vi "Convert_TrajectoryFile_To_PathWeaverJSON.vi"() -> ()   [LabVIEW 2019]
uses:
  <vilib>/Rock Robotics/WPI/ThirdParty/JAS_Junk/TrajLib/TypeDef/TRAJ_STATE.ctl
  <vilib>/Rock Robotics/WPI/ThirdParty/JAS_Junk/TrajLib/TypeDef/POSE2D.ctl
  <vilib>/Rock Robotics/WPI/ThirdParty/JAS_Junk/TrajLib/TypeDef/TRANSLATION2D.ctl
  <vilib>/Rock Robotics/WPI/ThirdParty/JAS_Junk/TrajLib/TypeDef/ROTATION2D.ctl
  <vilib>/Rock Robotics/WPI/ThirdParty/JAS_Junk/TrajLib/Trajectory_Library.lvlib
panel:
  in  "End Program":bool
  in  "Tab Control":T1(tab)
  in  "Trajectory CSV File":path
  in  "Read JSON Fiile":bool
  out "File Read Error":errorcluster
  in  "WheelBase":dbl=0.6
  out "Position":cluster{dbl[], dbl[]}[](graph)
  out "Trajectory Data":cluster{dbl[], dbl[]}[](graph)
  out "Traj States\nSize":i32
  out "Trajectory States":T2[](array[typedef]) {"POSE"."ROTATION"."SIN" format="%13.4f"; "POSE"."ROTATION"."COS" format="%13.4f"; "POSE"."ROTATION"."VALUE" format="%13.4f"; "POSE"."TRANSLATION"."Y" format="%14.3f"; "POSE"."TRANSLATION"."X" format="%14.3f"}
  in  "PathWeaver Length Units":T6(radio)
  out "File Saved\nWithout\nError":bool
  in  "Trajectory Type":enum32{"Radio Selection 1", "Radio Selection 2"}(radio)
  out "File Creation\nError":errorcluster
  in  "PathWeaver JSON File Name":path
  in  "CreateCmdList":bool
  out "Ready to\nWrite FIle":bool
  # "Convert trajectory CSV file to Pathweaver JSON file"
  # "Instructions: \n---------------- \nThis utility reads a trajectory CSV file,  The results are plotted for review.  \nThis file can then be written to a PathWeaver JSON file.\n\nNotes:\n---------\n - Pathweaver sets the Y orign at the top left.  This trajectory library utilties use the bottom right.  This utility converts the Y position value to be consistent. \n   There are no consequences when the trajectory is saved as a robot relative trajectory.  For absolute trajectories, the robot position needs to\n   condier this."
  # "Meters"
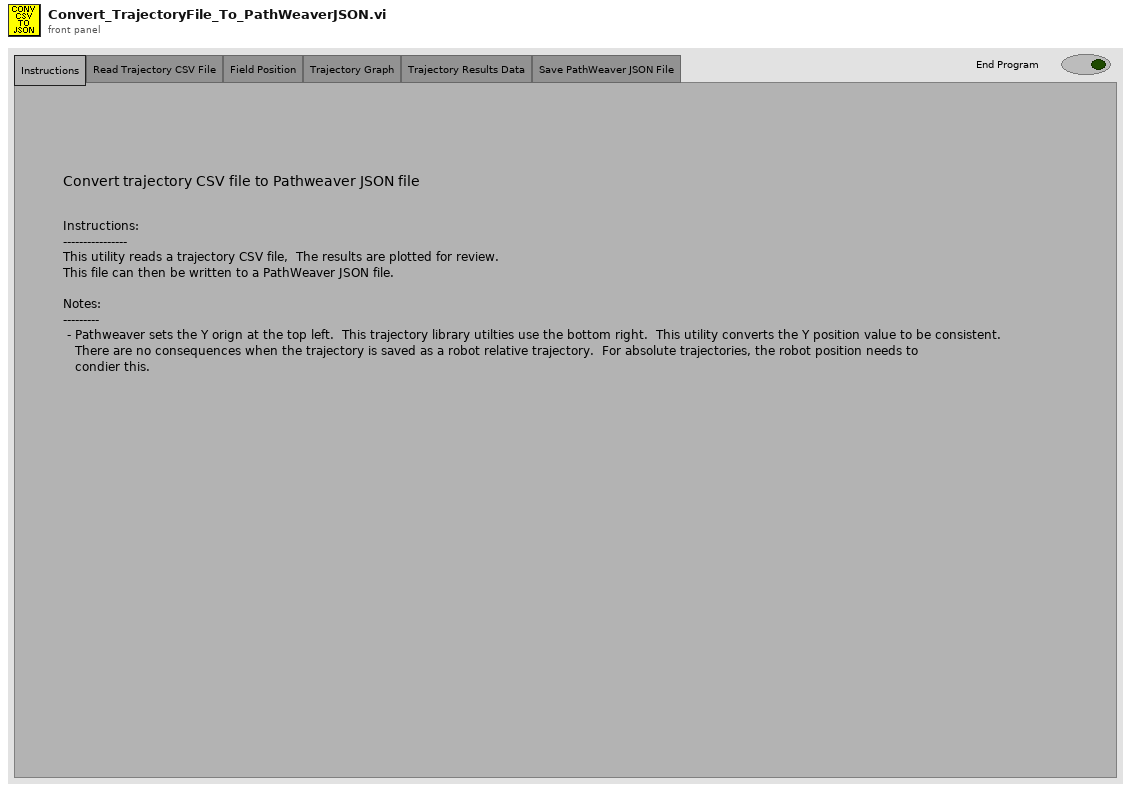
[diagram p1: front panel]
types:
  T1 = enum32{"Instructions", "Read Trajectory CSV File", "Field Position", "Trajectory Graph", "Trajectory Results Data", "Save PathWeaver JSON File"}
  T2 = typedef "Trajectory_Library.lvlib/TRAJ_STATE.ctl" = cluster{"TimeSeconds":dbl, "Velocity":dbl, "Acceleration":dbl, "POSE":T3, "Curvature":dbl}
  T3 = typedef "Trajectory_Library.lvlib/POSE2D.ctl" = cluster{"TRANSLATION":T4, "ROTATION":T5}
  T4 = typedef "Trajectory_Library.lvlib/TRANSLATION2D.ctl" = cluster{"X":dbl, "Y":dbl}
  T5 = typedef "Trajectory_Library.lvlib/ROTATION2D.ctl" = cluster{"VALUE":dbl, "COS":dbl, "SIN":dbl}
  T6 = enum32{"Radio Selection 1", "Radio Selection 2", "Radio Selection 3", "Radio Selection 4", "Radio Selection 5"}
  T7 = typedef "Trajectory_Library.lvlib/TRAJECTORY.ctl" = cluster{"TotalTImeSecs":dbl, "States":T2[]}
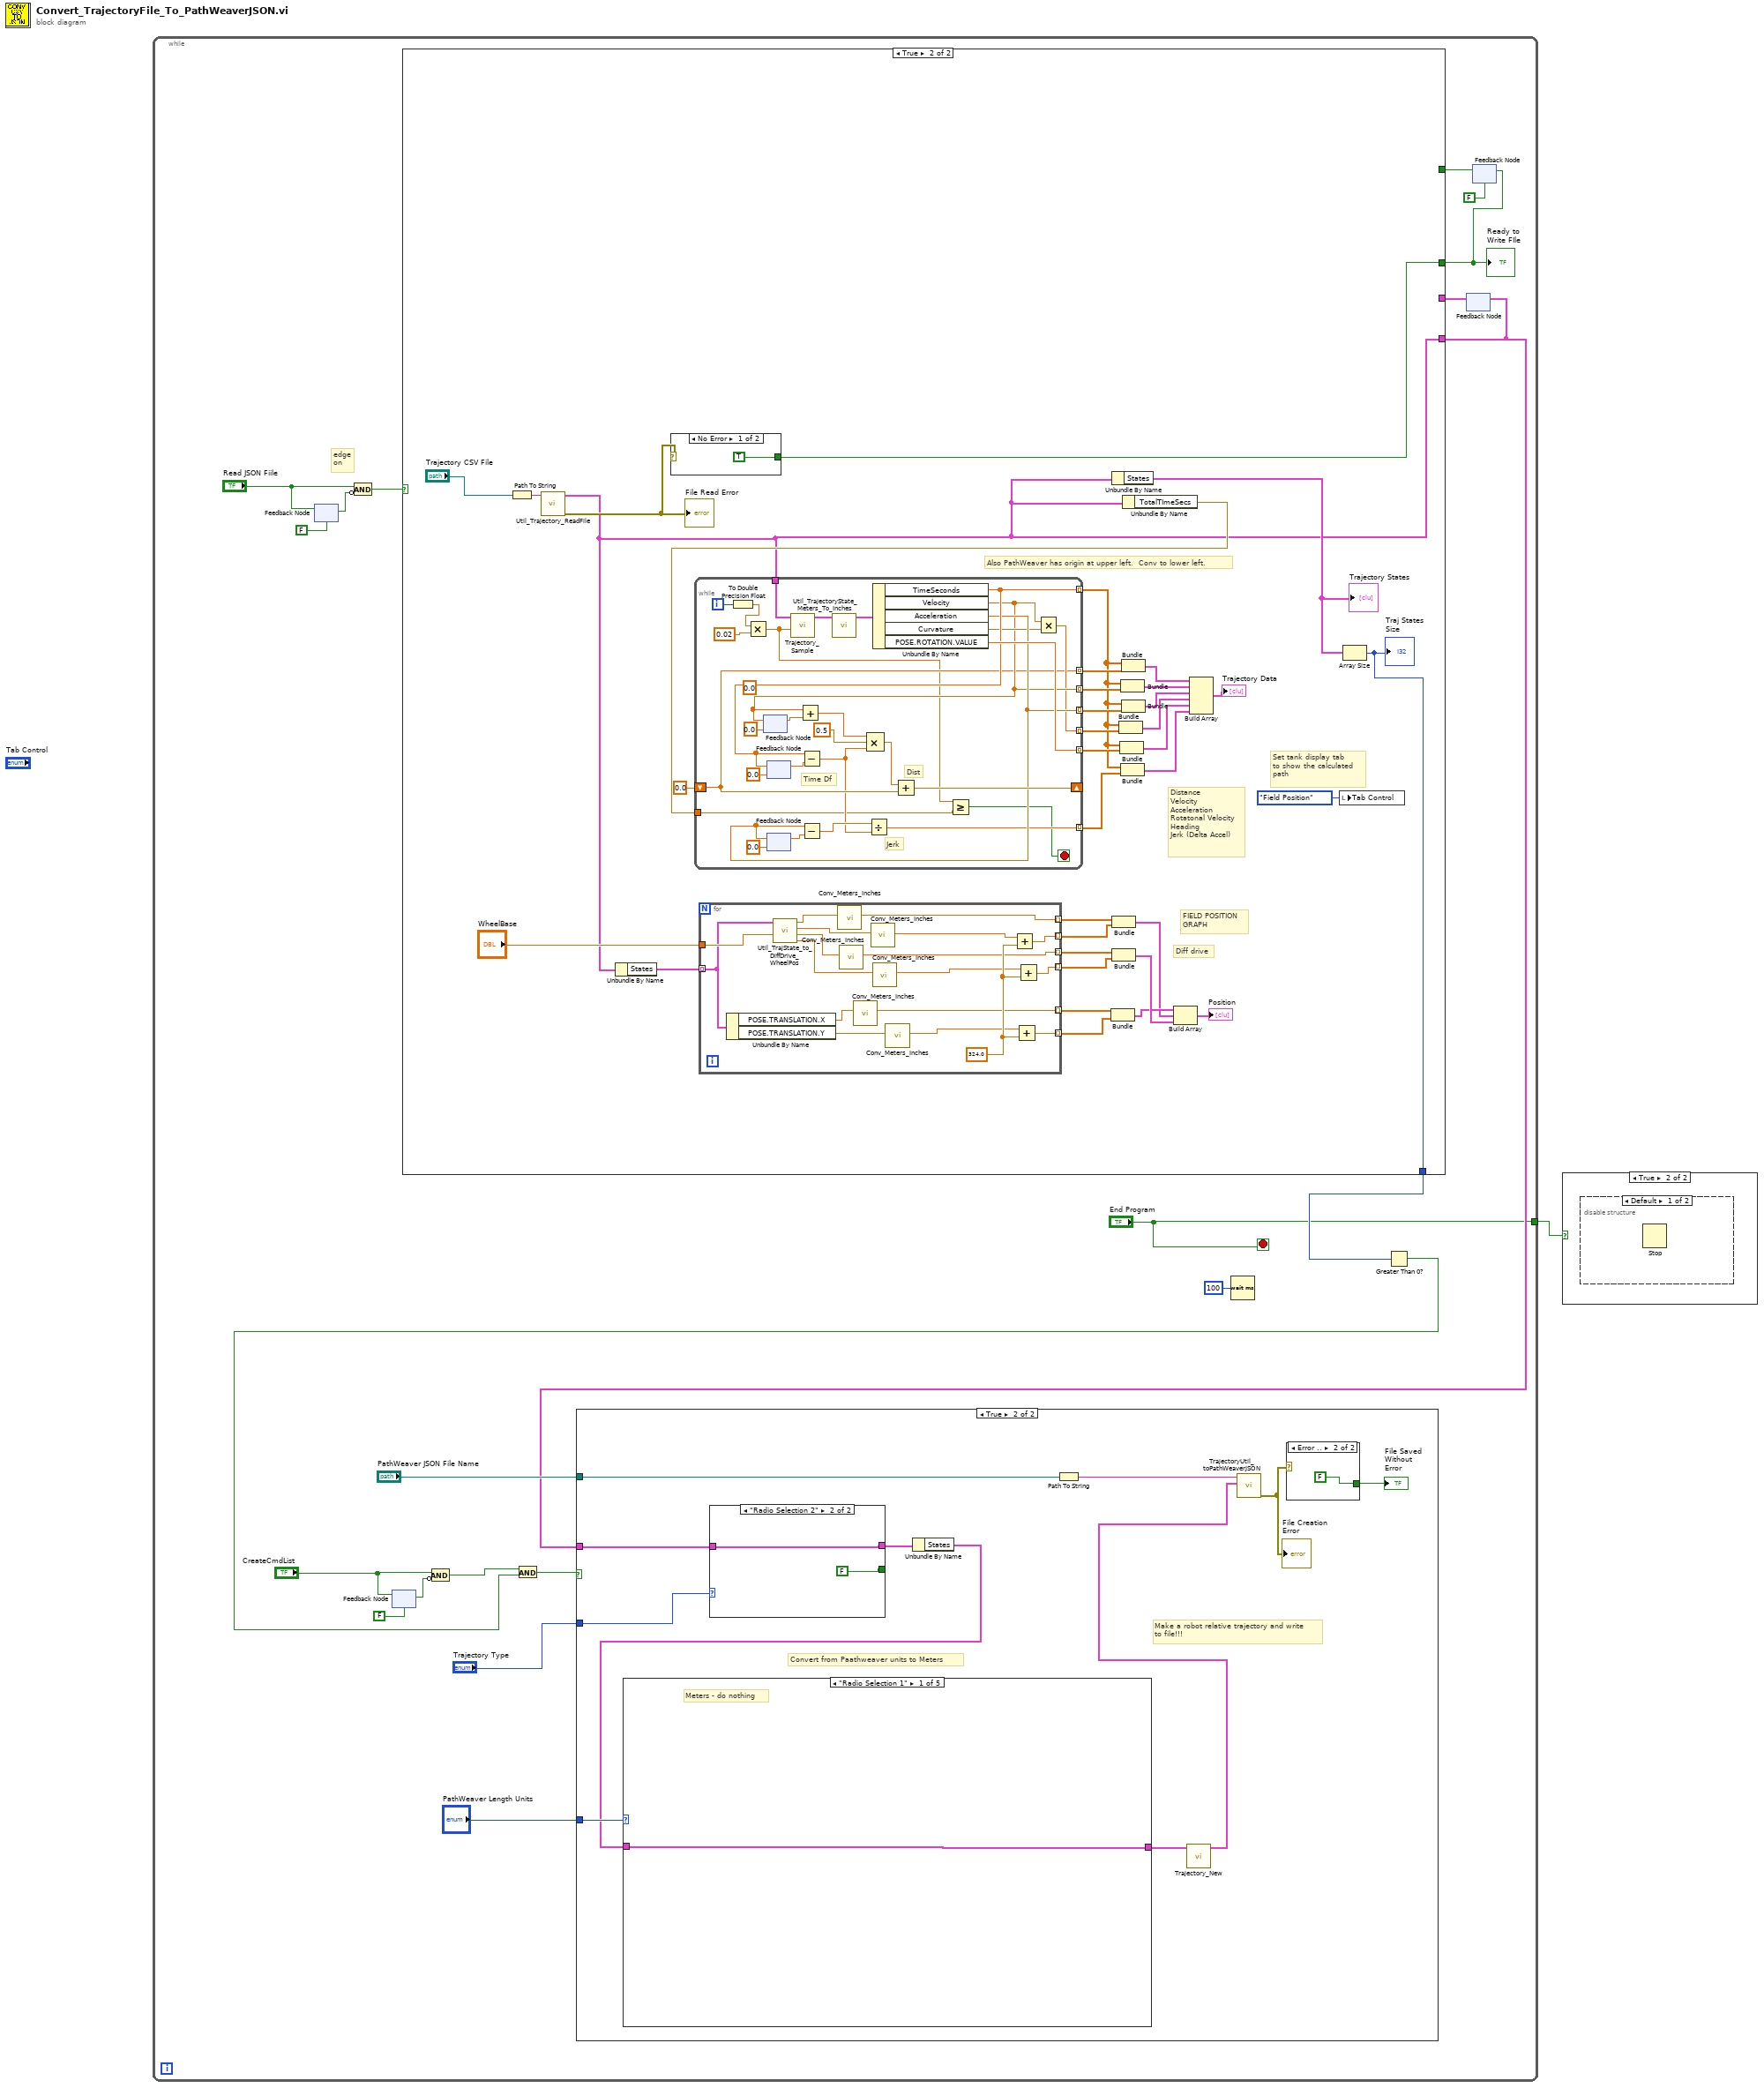
[diagram p0: block diagram]
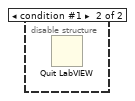
[diagram p3: hidden frame]
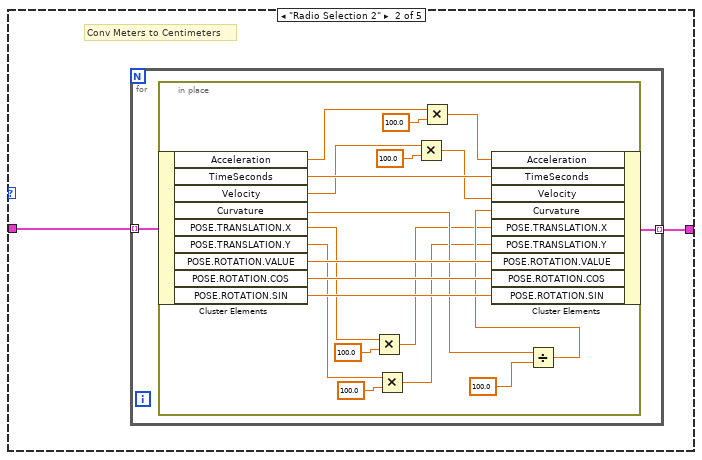
[diagram p5: hidden frame]
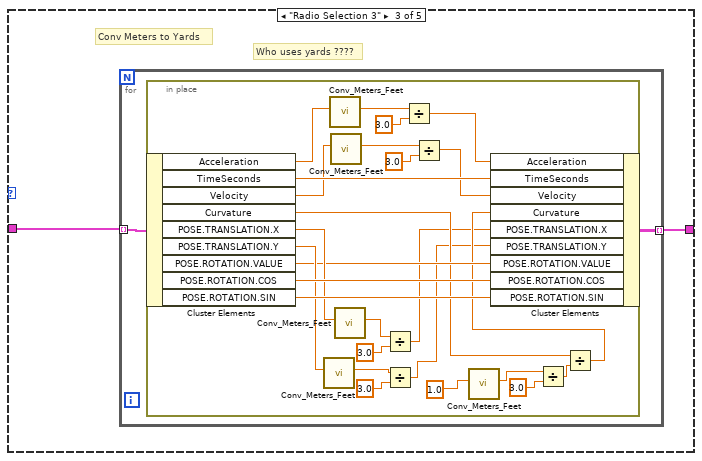
[diagram p6: hidden frame]
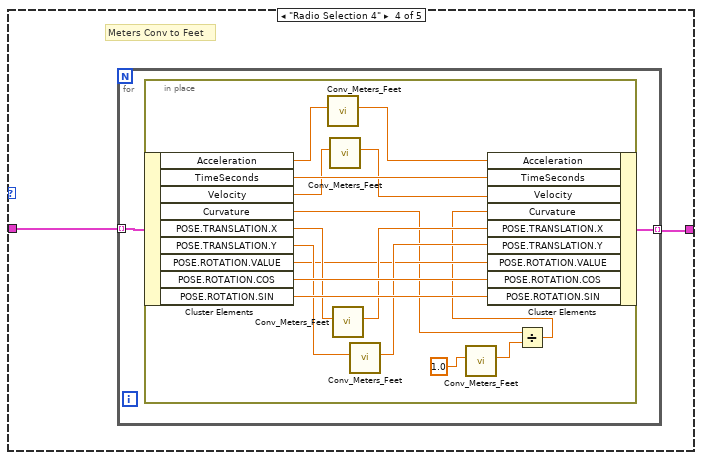
[diagram p7: hidden frame]
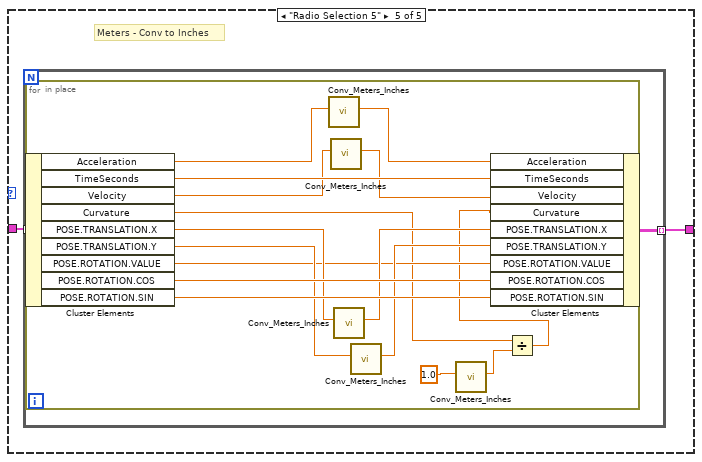
[diagram p8: hidden frame]
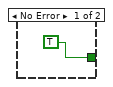
[diagram p9: hidden frame]
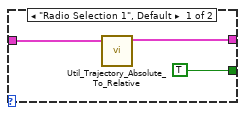
[diagram p10: hidden frame]
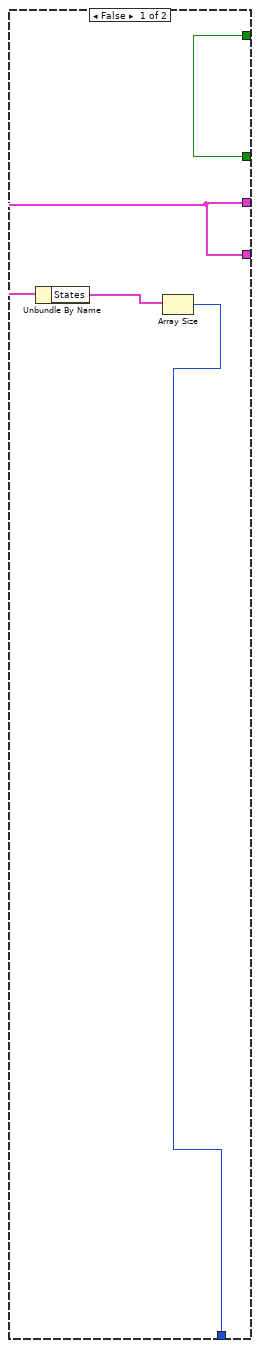
[diagram p11: hidden frame]
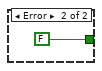
[diagram p12: hidden frame]
diagram:
  n1 = while {
    tunnel: ["End Program"] -> w1
    stop <- "End Program" stop-if-true
    # "edge\non"
    n2 = feedback #1(FALSE ("CreateCmdList")) -> (w12:bool)
    n3 = feedback-in #1("Read JSON Fiile") -> ()
    n4 = Compound Arithmetic op=AND("Read JSON Fiile", invert w12) -> (w10:bool)
    n5 = feedback-in #2("CreateCmdList") -> ()
    n6 = feedback #2(FALSE ("CreateCmdList")) -> (w15:bool)
    n7 = Compound Arithmetic op=AND("CreateCmdList", invert w15) -> (w14:bool)
    n8 = Wait (ms)(milliseconds to wait=u32 100) -> ()  [unwired: 1 out]
    n9 = feedback #3() -> (w21:T7)  [unwired: 1 in]
    n10 = feedback #4(FALSE) -> (w6:bool)
    n11 = case shown="True" w10 {
      tunnel: [w136 w139] -> w18
      tunnel: w21 -> [w136 _]
      tunnel: [w138 w174] -> w17
      tunnel: [w137 w172] -> w8
      tunnel: w6 -> [w137 _]
      frame False {
        n12 = Unbundle By Name(w136) -> ("States"=w135:T2[])
        n13 = Array Size(array=w135) -> (size(s)=w138:i32)
      }
      frame True {
        (unwired) 0.0
        # "Diff drive"
        # "FIELD POSITION\nGRAPH"
        # "Distance\nVelocity\nAcceleration\nRotatonal Velocity\nHeading\nJerk (Delta Accel)"
        # "Also PathWeaver has origin at upper left.  Conv to lower left."
        # "Set tank display tab\nto show the calculated\npath"
        n14 = Path To String(path="Trajectory CSV File") -> (string=w144:string)
        n15 = call <vilib>:"Util_Trajectory_ReadFile.vi"("FileName"=w144) -> ("error out"=w143:errorcluster, "outTRAJECTORY"=w139:T7)  [unwired: 8 in, 1 out]
        "File Read Error" <- w143
        n16 = Unbundle By Name(w139) -> ("States"=w145:T2[])
        n17 = case shown="No Error" w143 {
          tunnel: [TRUE FALSE] -> w172
          frame No Error {
          }
          frame Error {
          }
        }
        n18 = for {
          tunnel: w145 -> [w187] mode=indexing
          tunnel: "WheelBase" -> [w192]
          tunnel: [w181] -> w154 mode=indexing
          tunnel: [w183] -> w153 mode=indexing
          tunnel: [w179] -> w152 mode=indexing
          tunnel: [w182] -> w151 mode=indexing
          tunnel: [w176] -> w147 mode=indexing
          tunnel: [w177] -> w146 mode=indexing
          w184 = 324.0 ("y")
          n19 = Unbundle By Name(w187) -> ("POSE.TRANSLATION.X"=w186:dbl, "POSE.TRANSLATION.Y"=w185:dbl)
          n20 = call <vilib>:"Util_TrajState_to_DiffDrive_WheelPos.vi"("Wheelbase"=w192, "TRAJ_STATE"=w187) -> ("Right Y"=w188:dbl, "Right X"=w189:dbl, "Left Y"=w190:dbl, "Left X"=w191:dbl)  [unwired: 6 in]
          n21 = call <vilib>:"Conv_Meters_Inches.vi"("Meters"=w191) -> ("Inches"=w181:dbl)  [unwired: 10 in]
          n22 = call <vilib>:"Conv_Meters_Inches.vi"("Meters"=w189) -> ("Inches"=w179:dbl)  [unwired: 10 in]
          n23 = call <vilib>:"Conv_Meters_Inches.vi"("Meters"=w186) -> ("Inches"=w177:dbl)  [unwired: 10 in]
          n24 = call <vilib>:"Conv_Meters_Inches.vi"("Meters"=w190) -> ("Inches"=w180:dbl)  [unwired: 10 in]
          n25 = call <vilib>:"Conv_Meters_Inches.vi"("Meters"=w188) -> ("Inches"=w178:dbl)  [unwired: 10 in]
          n26 = call <vilib>:"Conv_Meters_Inches.vi"("Meters"=w185) -> ("Inches"=w175:dbl)  [unwired: 10 in]
          n27 = Add(x=w180, y=w184) -> (x+y=w183:dbl)
          n28 = Add(x=w175, y=w184) -> (x+y=w176:dbl)
          n29 = Add(x=w178, y=w184) -> (x+y=w182:dbl)
        }
        n30 = Bundle(w146, w147) -> (w149:cluster{dbl[], dbl[]})  [unwired: 1 in]
        n31 = Unbundle By Name(w139) -> ("States"=w140:T2[])
        "Trajectory States" <- w140
        n32 = Bundle(w154, w153) -> (w148:cluster{dbl[], dbl[]})  [unwired: 1 in]
        n33 = Bundle(w152, w151) -> (w150:cluster{dbl[], dbl[]})  [unwired: 1 in]
        n34 = Unbundle By Name(w139) -> ("TotalTImeSecs"=w156:dbl)
        n35 = while {
          tunnel: [w214] -> w158 mode=indexing
          tunnel: [w205] -> w168 mode=indexing
          tunnel: [w207] -> w167 mode=indexing
          tunnel: [w211] -> w166 mode=indexing
          tunnel: [w206] -> w165 mode=indexing
          tunnel: [w221] -> w164 mode=indexing
          shift-right: [w215] -> _
          shift-left: 0.0 -> [w205]
          tunnel: [w209] -> w157 mode=indexing
          tunnel: w156 -> [w201]
          tunnel: w139 -> [w199]
          i -> [w198]
          stop <- w200 stop-if-true
          # "Time Df"
          # "Jerk"
          # "Dist"
          n36 = To Double Precision Float(number=w198) -> (double precision float=w197:dbl)
          n37 = Multiply(x=w197, y=0.02) -> (x*y=w195:dbl)
          n38 = feedback #5(0.0 ("TimeSeconds")) -> (w217:dbl)
          n39 = feedback #6(0.0 ("TimeSeconds")) -> (w219:dbl)
          n40 = feedback #7(0.0 ("TimeSeconds")) -> (w212:dbl)
          n41 = call <vilib>:"Trajectory_Sample.vi"("Time"=w195, "InputTRAJECTORY"=w199) -> ("OutputTRAJ_STATE"=w193:T2)  [unwired: 9 in]
          n42 = call <vilib>:"Util_TrajectoryState_Meters_To_Inches.vi"("absTRAJECTORY"=w193) -> ("outputRelativeTRAJECTORY"=w194:T2)  [unwired: 10 in]
          n43 = Unbundle By Name(w194) -> ("TimeSeconds"=w214:dbl, "Velocity"=w207:dbl, "Acceleration"=w211:dbl, "Curvature"=w208:dbl, "POSE.ROTATION.VALUE"=w221:dbl)
          n44 = feedback-in #5(w207) -> ()
          n45 = feedback-in #6(w214) -> ()
          n46 = feedback-in #7(w211) -> ()
          n47 = Add(x=w207, y=w217) -> (x+y=w216:dbl)
          n48 = Subtract(x=w214, y=w219) -> (x-y=w202:dbl)
          n49 = Subtract(x=w211, y=w212) -> (x-y=w210:dbl)
          n50 = Compound Arithmetic op=MULTIPLY(w216, 0.5 ("value"), w202) -> (w204:dbl)
          n51 = Divide(x=w210, y=w202) -> (x/y=w209:dbl)
          n52 = Add(x=w204, y=w205) -> (x+y=w215:dbl)
          n53 = Greater Or Equal?(x=w195, y=w201) -> (x >= y?=w200:bool)
          n54 = Multiply(x=w207, y=w208) -> (x*y=w206:dbl)
        }
        n55 = Bundle(w158, w165) -> (w163:cluster{dbl[], dbl[]})  [unwired: 1 in]
        n56 = Bundle(w158, w164) -> (w162:cluster{dbl[], dbl[]})  [unwired: 1 in]
        n57 = Bundle(w158, w167) -> (w170:cluster{dbl[], dbl[]})  [unwired: 1 in]
        n58 = Bundle(w158, w157) -> (w159:cluster{dbl[], dbl[]})  [unwired: 1 in]
        n59 = Bundle(w158, w168) -> (w171:cluster{dbl[], dbl[]})  [unwired: 1 in]
        n60 = Bundle(w158, w166) -> (w169:cluster{dbl[], dbl[]})  [unwired: 1 in]
        n61 = Build Array(w149, w148, w150) -> (→"Position":cluster{dbl[], dbl[]}[])
        n62 = Build Array(w171, w170, w169, w163, w162, w159) -> (→"Trajectory Data":cluster{dbl[], dbl[]}[])
        n63 = local write "Tab Control"(T1."Field Position" ("Tab Control")) -> ()
        n64 = Array Size(array=w140) -> (size(s)=w174:i32)
        "Traj States\nSize" <- w174
      }
    }
    "Ready to\nWrite FIle" <- w8
    n65 = Greater Than 0?(x=w17) -> (x > 0?=w3:bool)
    n66 = And(x=w14, y=w3) -> (x .and. y?=w19:bool)
    n67 = case shown="True" w19 {
      tunnel: "PathWeaver JSON File Name" -> [_ w24]
      tunnel: w18 -> [_ w30]
      tunnel: "Trajectory Type" -> [_ w33]
      tunnel: "PathWeaver Length Units" -> [_ w31]
      frame False {
      }
      frame True {
        # "Convert from Paathweaver units to Meters"
        # "Make a robot relative trajectory and write\nto file!!!"
        n68 = case shown="\"Radio Selection 2\"" w33 {
          tunnel: w30 -> [w132 w134]
          tunnel: [w131 w134] -> w29
          tunnel: [TRUE FALSE] -> _
          frame "Radio Selection 1", Default {
            n69 = call <vilib>:"Util_Trajectory_Absolute_To_Relative.vi"("absTRAJECTORY"=w132) -> ("outputRelativeTRAJECTORY"=w131:T7)  [unwired: 10 in]
          }
          frame "Radio Selection 2" {
          }
        }
        n70 = Unbundle By Name(w29) -> ("States"=w28:T2[])
        n71 = case shown="\"Radio Selection 1\"" w31 {
          tunnel: w28 -> [w34 w35 w59 w89 w109]
          tunnel: [w34 w36 w58 w88 w108] -> w27
          frame "Radio Selection 1" {
            # "Meters - do nothing"
          }
          frame "Radio Selection 2" {
            # "Conv Meters to Centimeters"
            n72 = for {
              tunnel: w35 -> [w38] mode=indexing
              tunnel: [w37] -> w36 mode=indexing
              n73 = in-place {
                n74 = in-place-cluster #8(w38) -> ("Acceleration"=w49:dbl, "TimeSeconds"=w57:dbl, "Velocity"=w47:dbl, "Curvature"=w52:dbl, "POSE.TRANSLATION.X"=w39:dbl, "POSE.TRANSLATION.Y"=w43:dbl, "POSE.ROTATION.VALUE"=w54:dbl, "POSE.ROTATION.COS"=w56:dbl, "POSE.ROTATION.SIN"=w55:dbl)
                n75 = Multiply(x=w39, y=100.0) -> (x*y=w40:dbl)
                n76 = Multiply(x=w43, y=100.0) -> (x*y=w42:dbl)
                n77 = Multiply(x=w47, y=100.0) -> (x*y=w46:dbl)
                n78 = Multiply(x=w49, y=100.0) -> (x*y=w50:dbl)
                n79 = Divide(x=w52, y=100.0 ("Centimeter")) -> (x/y=w53:dbl)
                n80 = in-place-cluster #8("Acceleration"=w50, "TimeSeconds"=w57, "Velocity"=w46, "Curvature"=w53, "POSE.TRANSLATION.X"=w40, "POSE.TRANSLATION.Y"=w42, "POSE.ROTATION.VALUE"=w54, "POSE.ROTATION.COS"=w56, "POSE.ROTATION.SIN"=w55) -> (w37:T2)
              }
            }
          }
          frame "Radio Selection 3" {
            # "Who uses yards ????"
            # "Conv Meters to Yards"
            n81 = for {
              tunnel: w59 -> [w61] mode=indexing
              tunnel: [w60] -> w58 mode=indexing
              n82 = in-place {
                n83 = in-place-cluster #9(w61) -> ("Acceleration"=w81:dbl, "TimeSeconds"=w87:dbl, "Velocity"=w82:dbl, "Curvature"=w79:dbl, "POSE.TRANSLATION.X"=w83:dbl, "POSE.TRANSLATION.Y"=w84:dbl, "POSE.ROTATION.VALUE"=w80:dbl, "POSE.ROTATION.COS"=w86:dbl, "POSE.ROTATION.SIN"=w85:dbl)
                n84 = call <vilib>:"Conv_Meters_Feet.vi"("Meters"=w84) -> ("Feet"=w66:dbl)  [unwired: 10 in]
                n85 = call <vilib>:"Conv_Meters_Feet.vi"("Meters"=w81) -> ("Feet"=w76:dbl)  [unwired: 10 in]
                n86 = call <vilib>:"Conv_Meters_Feet.vi"("Meters"=w82) -> ("Feet"=w72:dbl)  [unwired: 10 in]
                n87 = call <vilib>:"Conv_Meters_Feet.vi"("Meters"=w83) -> ("Feet"=w63:dbl)  [unwired: 10 in]
                n88 = Divide(x=w63, y=3.0) -> (x/y=w62:dbl)
                n89 = Divide(x=w66, y=3.0) -> (x/y=w65:dbl)
                n90 = Divide(x=w76, y=3.0) -> (x/y=w74:dbl)
                n91 = Divide(x=w72, y=3.0) -> (x/y=w71:dbl)
                n92 = call <vilib>:"Conv_Meters_Feet.vi"("Meters"=1.0 ("Centimeter")) -> ("Feet"=w68:dbl)  [unwired: 10 in]
                n93 = Divide(x=w68, y=3.0) -> (x/y=w69:dbl)
                n94 = Divide(x=w79, y=w69) -> (x/y=w78:dbl)
                n95 = in-place-cluster #9("Acceleration"=w74, "TimeSeconds"=w87, "Velocity"=w71, "Curvature"=w78, "POSE.TRANSLATION.X"=w62, "POSE.TRANSLATION.Y"=w65, "POSE.ROTATION.VALUE"=w80, "POSE.ROTATION.COS"=w86, "POSE.ROTATION.SIN"=w85) -> (w60:T2)
              }
            }
          }
          frame "Radio Selection 4" {
            # "Meters Conv to Feet"
            n96 = for {
              tunnel: w89 -> [w91] mode=indexing
              tunnel: [w90] -> w88 mode=indexing
              n97 = in-place {
                n98 = in-place-cluster #10(w91) -> ("Acceleration"=w99:dbl, "TimeSeconds"=w107:dbl, "Velocity"=w101:dbl, "Curvature"=w93:dbl, "POSE.TRANSLATION.X"=w103:dbl, "POSE.TRANSLATION.Y"=w104:dbl, "POSE.ROTATION.VALUE"=w96:dbl, "POSE.ROTATION.COS"=w106:dbl, "POSE.ROTATION.SIN"=w105:dbl)
                n99 = call <vilib>:"Conv_Meters_Feet.vi"("Meters"=w99) -> ("Feet"=w98:dbl)  [unwired: 10 in]
                n100 = call <vilib>:"Conv_Meters_Feet.vi"("Meters"=w101) -> ("Feet"=w100:dbl)  [unwired: 10 in]
                n101 = call <vilib>:"Conv_Meters_Feet.vi"("Meters"=w103) -> ("Feet"=w102:dbl)  [unwired: 10 in]
                n102 = call <vilib>:"Conv_Meters_Feet.vi"("Meters"=w104) -> ("Feet"=w97:dbl)  [unwired: 10 in]
                n103 = call <vilib>:"Conv_Meters_Feet.vi"("Meters"=1.0 ("Centimeter")) -> ("Feet"=w94:dbl)  [unwired: 10 in]
                n104 = Divide(x=w93, y=w94) -> (x/y=w92:dbl)
                n105 = in-place-cluster #10("Acceleration"=w98, "TimeSeconds"=w107, "Velocity"=w100, "Curvature"=w92, "POSE.TRANSLATION.X"=w102, "POSE.TRANSLATION.Y"=w97, "POSE.ROTATION.VALUE"=w96, "POSE.ROTATION.COS"=w106, "POSE.ROTATION.SIN"=w105) -> (w90:T2)
              }
            }
          }
          frame "Radio Selection 5" {
            # "Meters - Conv to Inches"
            n106 = for {
              tunnel: w109 -> [w111] mode=indexing
              tunnel: [w110] -> w108 mode=indexing
              n107 = in-place {
                n108 = in-place-cluster #11(w111) -> ("Acceleration"=w119:dbl, "TimeSeconds"=w127:dbl, "Velocity"=w121:dbl, "Curvature"=w113:dbl, "POSE.TRANSLATION.X"=w123:dbl, "POSE.TRANSLATION.Y"=w124:dbl, "POSE.ROTATION.VALUE"=w116:dbl, "POSE.ROTATION.COS"=w126:dbl, "POSE.ROTATION.SIN"=w125:dbl)
                n109 = call <vilib>:"Conv_Meters_Inches.vi"("Meters"=w119) -> ("Inches"=w118:dbl)  [unwired: 10 in]
                n110 = call <vilib>:"Conv_Meters_Inches.vi"("Meters"=w121) -> ("Inches"=w120:dbl)  [unwired: 10 in]
                n111 = call <vilib>:"Conv_Meters_Inches.vi"("Meters"=w123) -> ("Inches"=w122:dbl)  [unwired: 10 in]
                n112 = call <vilib>:"Conv_Meters_Inches.vi"("Meters"=w124) -> ("Inches"=w117:dbl)  [unwired: 10 in]
                n113 = call <vilib>:"Conv_Meters_Inches.vi"("Meters"=1.0 ("Centimeter")) -> ("Inches"=w114:dbl)  [unwired: 10 in]
                n114 = Divide(x=w113, y=w114) -> (x/y=w112:dbl)
                n115 = in-place-cluster #11("Acceleration"=w118, "TimeSeconds"=w127, "Velocity"=w120, "Curvature"=w112, "POSE.TRANSLATION.X"=w122, "POSE.TRANSLATION.Y"=w117, "POSE.ROTATION.VALUE"=w116, "POSE.ROTATION.COS"=w126, "POSE.ROTATION.SIN"=w125) -> (w110:T2)
              }
            }
          }
        }
        n116 = Path To String(path=w24) -> (string=w23:string)
        n117 = call <vilib>:"Trajectory_New.vi"("TRAJ_STATES"=w27) -> ("TRAJECTORY"=w26:T7)  [unwired: 10 in]
        n118 = call <vilib>:"TrajectoryUtil_toPathWeaverJSON.vi"("inTRAJECTORY"=w26, "FileName"=w23) -> ("error out"=w25:errorcluster)  [unwired: 8 in, 1 out]
        "File Creation\nError" <- w25
        n119 = case shown="Error .." w25 {
          tunnel: [TRUE ("File Saved\nWithout\nError") FALSE ("File Saved\nWithout\nError")] -> w32
          frame No Error {
          }
          frame Error {
          }
        }
        "File Saved\nWithout\nError" <- w32
      }
    }
    n120 = feedback-in #3(w18) -> ()
    n121 = feedback-in #4(w8) -> ()
  }
  n122 = case shown="True" w1 {
    frame False {
    }
    frame True {
      n123 = disable-structure shown="Default" {
        frame condition #0 (active) {
          n124 = Stop() -> ()  [unwired: 1 in]
        }
        frame condition #1 {
          n125 = Quit LabVIEW() -> ()  [unwired: 1 in]
        }
      }
    }
  }
